vi "serialWrite.vi"(8 "error in (no error)":errorcluster, 10 "text":string, 11 "Python":T1) -> (0 "error out":errorcluster, 2 "reply":string, 3 "Num loops":i32)   [LabVIEW 2022 SP3]
uses:
  PythonCtrl.ctl
  Processors.ctl
panel:
  out "appended array":i32[](array[numeric])
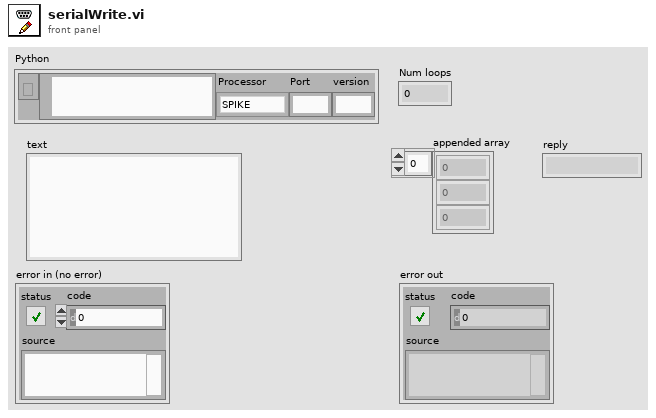
[diagram p1: front panel]
types:
  T1 = typedef "PythonCtrl.ctl" = cluster{"session":refnum<k35>, "PyPath":path, "Processor":T2, "Port":string, "version":string}
  T2 = typedef "Processors.ctl" = enum16{"SPIKE", "Pi", "Pi_ssh", "OpenMV", "Dunio"}
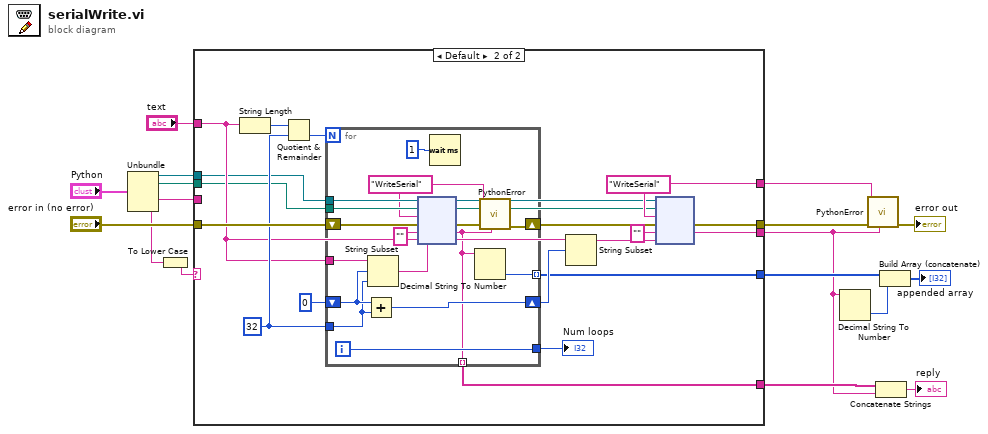
[diagram p0: block diagram]
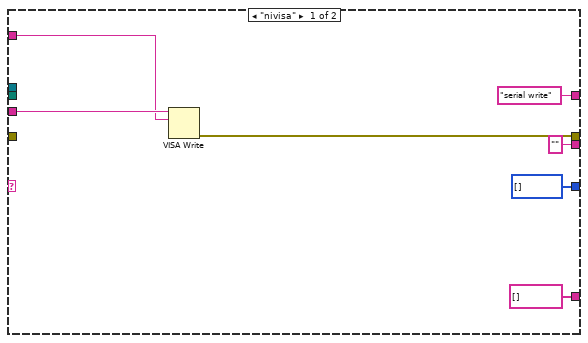
[diagram p2: hidden frame]
diagram:
  n1 = Unbundle("Python") -> ("session"=w16:refnum<k35>, "PyPath"=w17:path, "Port"=w1:string, "version"=w3:string)  [unwired: 1 out]
  n2 = To Lower Case(string=w3) -> (all lower case string=w2:string)
  n3 = case shown="Default" w2 {
    tunnel: w17 -> [_ w25]
    tunnel: w16 -> [_ w26]
    tunnel: "error in (no error)" -> [_ w39]
    tunnel: "text" -> [w23 w27]
    tunnel: [i32[] [] w33] -> w12
    tunnel: [w22 w32] -> w10
    tunnel: ["serial write" ("function name") w30] -> w7
    tunnel: [string[] [] w29] -> w6
    tunnel: ["" ("function name") w28] -> w5
    tunnel: w1 -> [w24 _]
    frame "nivisa" {
      n4 = VISA Write(VISA resource name=w24, write buffer=w23) -> (error out=w22:errorcluster)  [unwired: 1 in, 2 out]
    }
    frame Default {
      w30 = "WriteSerial" ("function name")
      w36 = 32 ("length (rest)")
      n5 = String Length(string=w27) -> (length=w37:i32)
      n6 = Quotient & Remainder(x=w37, y=w36) -> (floor(x/y)=w35:i32)  [unwired: 1 out]
      n7 = for {
        N: w35 -> [_]
        tunnel: w27 -> [w58]
        shift-right: [w56] -> w34
        shift-left: 0 -> [w57]
        tunnel: w36 -> [w55]
        tunnel: [w53] -> w42
        shift-right: [w47] -> w40
        shift-left: w39 -> [w51]
        tunnel: w26 -> [w50]
        tunnel: w25 -> [w49]
        tunnel: [w45] -> w33 mode=indexing
        tunnel: [w43] -> w29 mode=indexing
        i -> [w53]
        w44 = "WriteSerial" ("function name")
        n8 = Add(x=w57, y=w55) -> (x+y=w56:i32)
        n9 = String Subset(string=w58, offset (0)=w57, length (rest)=w55) -> (substring=w52:string)
        n10 = node(w50, w49, w44, w51, "" ("function name"), w52) -> (w48:errorcluster, w43:string)  [unwired: 1 in, 3 out]
        n11 = Wait (ms)(milliseconds to wait=u32 1) -> ()  [unwired: 1 out]
        n12 = Decimal String To Number(string=w43) -> (number=w45:i32)  [unwired: 2 in, 1 out]
        n13 = call "PythonError.vi"("reply"=w43, "error in (no error)"=w48, "function name"=w44) -> ("error out"=w47:errorcluster)  [unwired: 8 in]
      }
      "Num loops" <- w42
      n14 = String Subset(string=w27, offset (0)=w34) -> (substring=w41:string)  [unwired: 1 in]
      n15 = node(w26, w25, w30, w40, "" ("function name"), w41) -> (w32:errorcluster, w28:string)  [unwired: 1 in, 3 out]
    }
  }
  n16 = Decimal String To Number(string=w5) -> (number=w8:i32)  [unwired: 2 in, 1 out]
  n17 = call "PythonError.vi"("reply"=w5, "error in (no error)"=w10, "function name"=w7) -> ("error out"=→"error out":errorcluster)  [unwired: 8 in]
  n18 = Concatenate Strings(w6, w5) -> (→"reply":string)
  n19 = Build Array (concatenate)(w12, w8) -> (→"appended array":i32[])
